vi "Roller Latch 2.vi"(0 "Switch":bool) -> (1 "Output 1":bool, 2 "Output 2":bool)   [LabVIEW 2013]
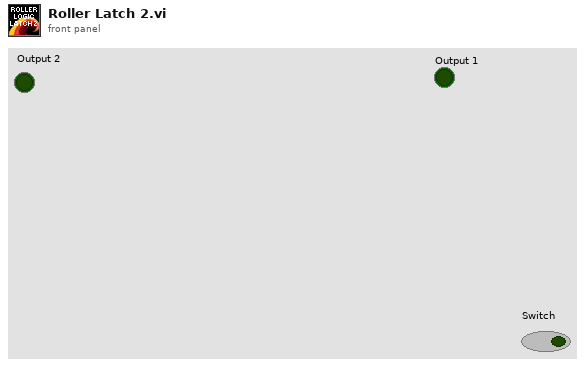
[diagram p1: front panel]
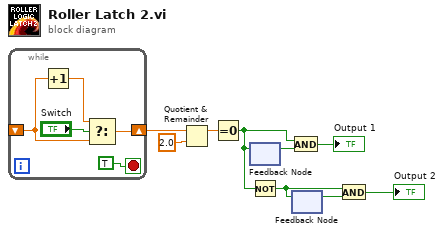
[diagram p0: block diagram]
diagram:
  n1 = while {
    shift-right: [w10] -> w4
    shift-left: _ -> [w13]
    stop <- TRUE stop-if-true
    n2 = Increment(x=w13) -> (x+1=w14:dbl)
    n3 = Select(t=w14, s="Switch", f=w13) -> (s? t:f=w10:dbl)
  }
  n4 = Quotient & Remainder(x=w4, y=2.0) -> (x-y*floor(x/y)=w3:dbl)  [unwired: 1 out]
  n5 = Equal To 0?(x=w3) -> (x = 0?=w2:bool)
  n6 = feedback #1() -> (w7:bool)  [unwired: 1 in]
  n7 = feedback-in #1(w2) -> ()
  n8 = Not(x=w2) -> (.not. x?=w1:bool)
  n9 = And(x=w2, y=w7) -> (x .and. y?=→"Output 1":bool)
  n10 = feedback-in #2(w1) -> ()
  n11 = feedback #2() -> (w8:bool)  [unwired: 1 in]
  n12 = And(x=w1, y=w8) -> (x .and. y?=→"Output 2":bool)
